vi "Tent Purge Toggle.vi"() -> ()   [LabVIEW 2016]
uses:
  <vilib>/DAQmx/write.llb/DAQmx Write (Digital Bool 1Line 1Point).vi
  <vilib>/DAQmx/miscellaneous.llb/DAQmx Fill In Error Info.vi
panel:
  out "?":bool
  in  "Permit Auto-on":bool
  in  "stop":bool
  out "Purging":bool
  in  "Tent Purge ON":bool
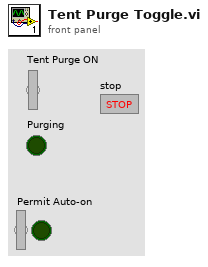
[diagram p1: front panel]
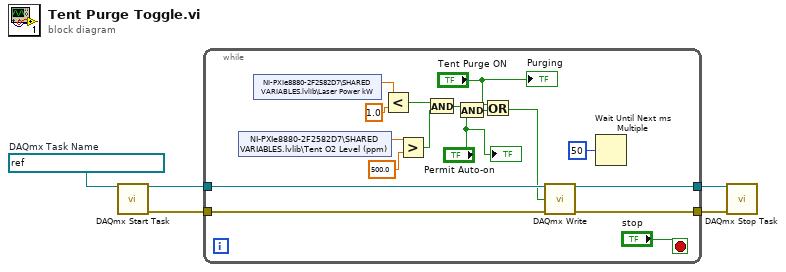
[diagram p0: block diagram]
diagram:
  w4 = refnum<k21> "Tent Purge Solenoid ON"  # DAQmx Task Name
  n1 = call <vilib>:"DAQmx Start Task.vi"("task/channels in"=w4) -> ("task out"=w5:refnum<k21>, "error out"=w2:errorcluster)  [unwired: 13 in]
  n2 = while {
    tunnel: w5 -> [w21]
    tunnel: [w19] -> w3
    tunnel: w2 -> [w20]
    tunnel: [w18] -> w1
    stop <- "stop" stop-if-true
    n3 = shared-variable "NI-PXIe8880-2F2582D7\\SHARED VARIABLES.lvlib\\Tent O2 Level (ppm)"() -> (w6:dbl)  [unwired: 1 in, 1 out]
    n4 = shared-variable "NI-PXIe8880-2F2582D7\\SHARED VARIABLES.lvlib\\Laser Power kW"() -> (w7:dbl)  [unwired: 1 in, 1 out]
    n5 = Less?(x=w7, y=1.0) -> (x < y?=w12:bool)
    n6 = Greater?(x=w6, y=500.0) -> (0:w11:bool)
    n7 = And(x=w12, y=w11) -> (x .and. y?=w10:bool)
    n8 = And(x=w10, y="Permit Auto-on") -> (x .and. y?=w9:bool)
    n9 = Or(x="Tent Purge ON", y=w9) -> (x .or. y?=w16:bool)
    n10 = call-poly <vilib>:"DAQmx Write.vi"("task/channels in"=w21, "data"=w16, "error in"=w20) -> ("task out"=w19:refnum<k21>, "error out"=w18:errorcluster)  [unwired: 10 in, 1 out]
    n11 = Wait Until Next ms Multiple(millisecond multiple=u32 50) -> ()  [unwired: 1 out]
    "Purging" <- "Tent Purge ON"
    "?" <- "Permit Auto-on"
  }
  n12 = call <vilib>:"DAQmx Stop Task.vi"("task/channels in"=w3, "error in"=w1) -> ()  [unwired: 12 in, 2 out]
